vi "Pre Launch Init.vi"(11 "Instrument Owner in":refnum<class "Instrument Owner.lvclass">) -> (0 "error out":errorcluster, 3 "Instrument Owner out":refnum<class "Instrument Owner.lvclass">)   [LabVIEW 2020, in "Instrument Handler.lvlib" / "Instrument Owner.lvclass"]
doc: "(<B>Filename</B>: Actor Framework.lvlib:Actor.lvclass:Pre Launch Init.vi)\n\nDefines behavior that occurs after the Launch Nested Actor method is invoked but before the actor's Actor Core method begins running.\n\nThis implementation populates the Sync DVR."
uses:
  Instrument Owner.lvclass
  C:/Current projects/WS/PPL/HDH.Actor Framework.Core.Actor.lvlibp/1abvi3w/vi.lib/ActorFramework/Actor/Actor.lvclass
  Instrument Owner.lvclass/Instrument Owner.ctl
  PPL/HDH.Actor Framework.Core.Sequencer.lvlibp/Sequencer/Sequencer.lvclass
  PPL/HDH.Data.Generic.lvlibp/Synchronization/Notifier/Notifier.lvclass
  PPL/HDH.Actor Framework.Core.Actor.lvlibp/1abvi3w/vi.lib/ActorFramework/Actor/Actor.lvclass
  C:/Current projects/WS/PPL/HDH.Actor Framework.Core.Sequencer.lvlibp/Sequencer/Sequencer.lvclass
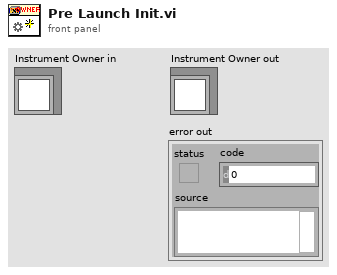
[diagram p1: front panel]
types:
  T1 = typedef "Instrument Handler.lvlib/Ctl_InstrumentSynchronicationCluster.ctl" = cluster{"Launched?":bool, "Driver Path":path, "Alias":string, "Connection Type":T2, "Pre Initialization Data":variant, "Enqueue Sync":refnum<class "Notifier.lvclass">, "Enqueue Lock":T3, "Owner Enqueuer":refnum<class "Message Enqueuer.lvclass">, "Owner":refnum<class "Sequencer Core.lvclass">, "Instrument ID":u32}
  T2 = typedef "HDH.Actor Framework.Core.Instrument Driver.lvlibp/Instrument Driver.lvclass/Ctl_ConnectionType.ctl" = enum16{"BuiltIn/System", "PXI/PCI", "USB", "GPIB", "VXI", "Serial", "TCP/IP", "cRIO", "SCXI", "cDAQ", "SwitchBlock", "SCC", "FireWire", "Accessory", "CAN", "SwitchBlock Device"}
  T3 = typedef "Semaphore RefNum" = refnum<k1>
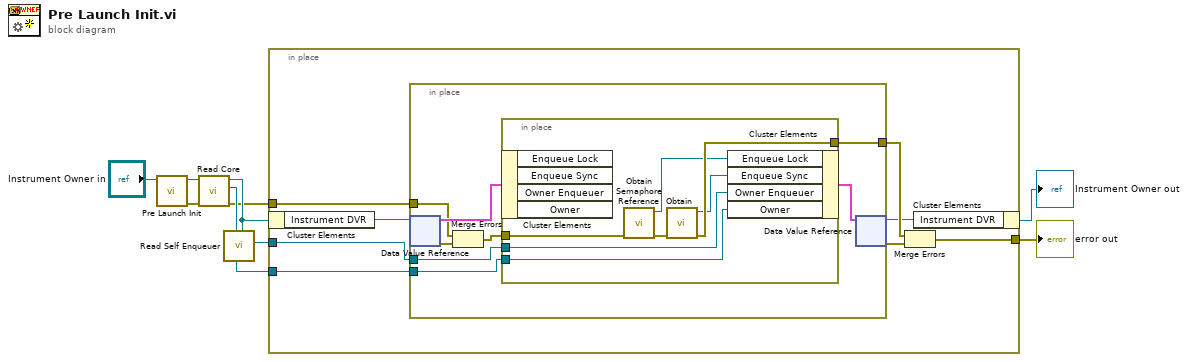
[diagram p0: block diagram]
diagram:
  n1 = call-parent "Pre Launch Init.vi"("Sequencer in"="Instrument Owner in") -> ("error out"=w8:errorcluster, "Sequencer out"=w6:refnum<class "Instrument Owner.lvclass">)  [unwired: 9 in]
  n2 = call "Read Core.vi"("error in (no error)"=w8, "Sequencer in"=w6) -> ("error out"=w2:errorcluster, "Core"=w3:refnum<class "Sequencer Core.lvclass">, "Sequencer out"=w4:refnum<class "Instrument Owner.lvclass">)  [unwired: 7 in]
  n3 = call "Read Self Enqueuer.vi"("Actor"=w4) -> ("Self Enqueuer"=w7:refnum<class "Message Enqueuer.lvclass">)  [unwired: 10 in]
  n4 = in-place {
    in-place-border: [w14] -> w9
    in-place-border: w7 -> [w12]
    in-place-border: w3 -> [w11]
    in-place-border: w2 -> [w10]
    n5 = in-place-cluster #1(w4) -> ("Instrument DVR"=w16:refnum<data-value>)
    n6 = in-place {
      in-place-border: [w25] -> w17
      in-place-border: w12 -> [w21]
      in-place-border: w11 -> [w20]
      in-place-border: w10 -> [w18]
      n7 = in-place-dvr #2(w16) -> (w24:T1, w22:errorcluster)
      n8 = Merge Errors(w18, w22) -> (w19:errorcluster)
      n9 = in-place {
        in-place-border: [w32] -> w25
        in-place-border: w19 -> [w30]
        in-place-border: w21 -> [w27]
        in-place-border: w20 -> [w26]
        n10 = in-place-cluster #3(w24) -> ()  [unwired: 4 out]
        n11 = call <vilib>:"Obtain Semaphore Reference.vi"("error in (no error)"=w30) -> ("error out"=w29:errorcluster, "semaphore"=w28:T3)  [unwired: 4 in, 1 out]
        n12 = call "Obtain.vi"("error in (no error)"=w29) -> ("error out"=w32:errorcluster, "Notifier out"=w31:refnum<class "Notifier.lvclass">)  [unwired: 8 in, 1 out]
        n13 = in-place-cluster #3("Enqueue Lock"=w28, "Enqueue Sync"=w31, "Owner Enqueuer"=w27, "Owner"=w26) -> (w23:T1)
      }
      n14 = in-place-dvr #2(w23) -> (w15:refnum<data-value>, w13:errorcluster)
    }
    n15 = Merge Errors(w17, w13) -> (w14:errorcluster)
    n16 = in-place-cluster #1("Instrument DVR"=w15) -> (→"Instrument Owner out":refnum<class "Instrument Owner.lvclass">)
  }
  "error out" <- w9
